vi "Handle Picture Key Down Event.vi"(7 "VKey":T1, 8 "error in (no error)":errorcluster, 11 "dialog info in":T2={"steering frame ref"=refnum, "active wheel indexes"=[], "FP Refs"={"VI Refnum"=refnum, "Menu Ref"=refnum, "Sub Panel"=refnum, "picture"=refnum, "Steering Type"=refnum, "zoom in"=refnum, "zoom out"=refnum, "zoom extents"=refnum, "Wheels"=refnum, "Add Wheel"=refnum, "Remove Wheel"=refnum, "Copy Wheel"=refnum, "Angle Units"=refnum}, "subpanel info"={"subpanel VI refs"=[], "subpanel types"=[], "main to subpanel command events"=[]}, "picture dragging state"={"dragging"=FALSE, "wheel index"=-1, "dragging mode"=enum."translate", "wheel start position"={"x"=0.0, "y"=0.0, "theta"=0.0}, "relative mouse position"={"x"=0.0, "y"=0.0}, "relative mouse init angle (rad)"=0.0}, "picture size (pixels)"={"Width"=500, "Height"=500}, "picture grid"=bytes[0], "click zones group"={"click zones array"=[], "num click zones"=0}, "draw options"={"draw wheel states?"=FALSE, "highlight wheel index"=-1, "pixels per unit"=10.0, "draw forward velocity?"=FALSE, "velocity scale"=1.0}}) -> (0 "error out":errorcluster, 1 "discard?":bool, 3 "dialog info out":T2={"steering frame ref"=refnum, "active wheel indexes"=[], "FP Refs"={"VI Refnum"=refnum, "Menu Ref"=refnum, "Sub Panel"=refnum, "picture"=refnum, "Steering Type"=refnum, "zoom in"=refnum, "zoom out"=refnum, "zoom extents"=refnum, "Wheels"=refnum, "Add Wheel"=refnum, "Remove Wheel"=refnum, "Copy Wheel"=refnum, "Angle Units"=refnum}, "subpanel info"={"subpanel VI refs"=[], "subpanel types"=[], "main to subpanel command events"=[]}, "picture dragging state"={"dragging"=FALSE, "wheel index"=-1, "dragging mode"=enum."translate", "wheel start position"={"x"=0.0, "y"=0.0, "theta"=0.0}, "relative mouse position"={"x"=0.0, "y"=0.0}, "relative mouse init angle (rad)"=0.0}, "picture size (pixels)"={"Width"=500, "Height"=500}, "picture grid"=bytes[0], "click zones group"={"click zones array"=[], "num click zones"=0}, "draw options"={"draw wheel states?"=FALSE, "highlight wheel index"=-1, "pixels per unit"=10.0, "draw forward velocity?"=FALSE, "velocity scale"=1.0}})   [LabVIEW 2017, in "NI_Robotics_Configure Steering Frame.lvlib"]
uses:
  <vilib>/robotics/Dialog/Configure Steering Frame/NI_Robotics_Configure Steering Frame.lvlib
  <vilib>/robotics/Dialog/Configure Steering Frame/Dialog Info.ctl
  <vilib>/robotics/Steering/Steering Frame/NI_Robotics_Steering Frame.lvclass
  <vilib>/robotics/Dialog/Configure Steering Frame/FP Refs.ctl
  <vilib>/robotics/Dialog/Configure Steering Frame/Subpanel Info.ctl
  <vilib>/robotics/Dialog/Configure Steering Frame/Main to Subpanel Command Event.ctl
  <vilib>/robotics/Dialog/Configure Steering Frame/Main to Subpanel Command.ctl
  <vilib>/robotics/Dialog/Configure Steering Frame/Dragging State.ctl
  <vilib>/robotics/Dialog/Configure Steering Frame/Dragging Mode.ctl
  <vilib>/Utility/miscctls.llb/LVBoundsTypeDef.ctl
  <vilib>/robotics/Dialog/Configure Steering Frame/Click Zone.ctl
  <vilib>/robotics/Utilities/Visualization/Steering Visualization/Steering Picture/Draw Steering Frame Options.ctl
  <vilib>/event_ctls.llb/eventvkey.ctl
  <vilib>/robotics/Utilities/Visualization/Steering Visualization/Steering Picture/NI_Robotics_Steering Picture.lvlib
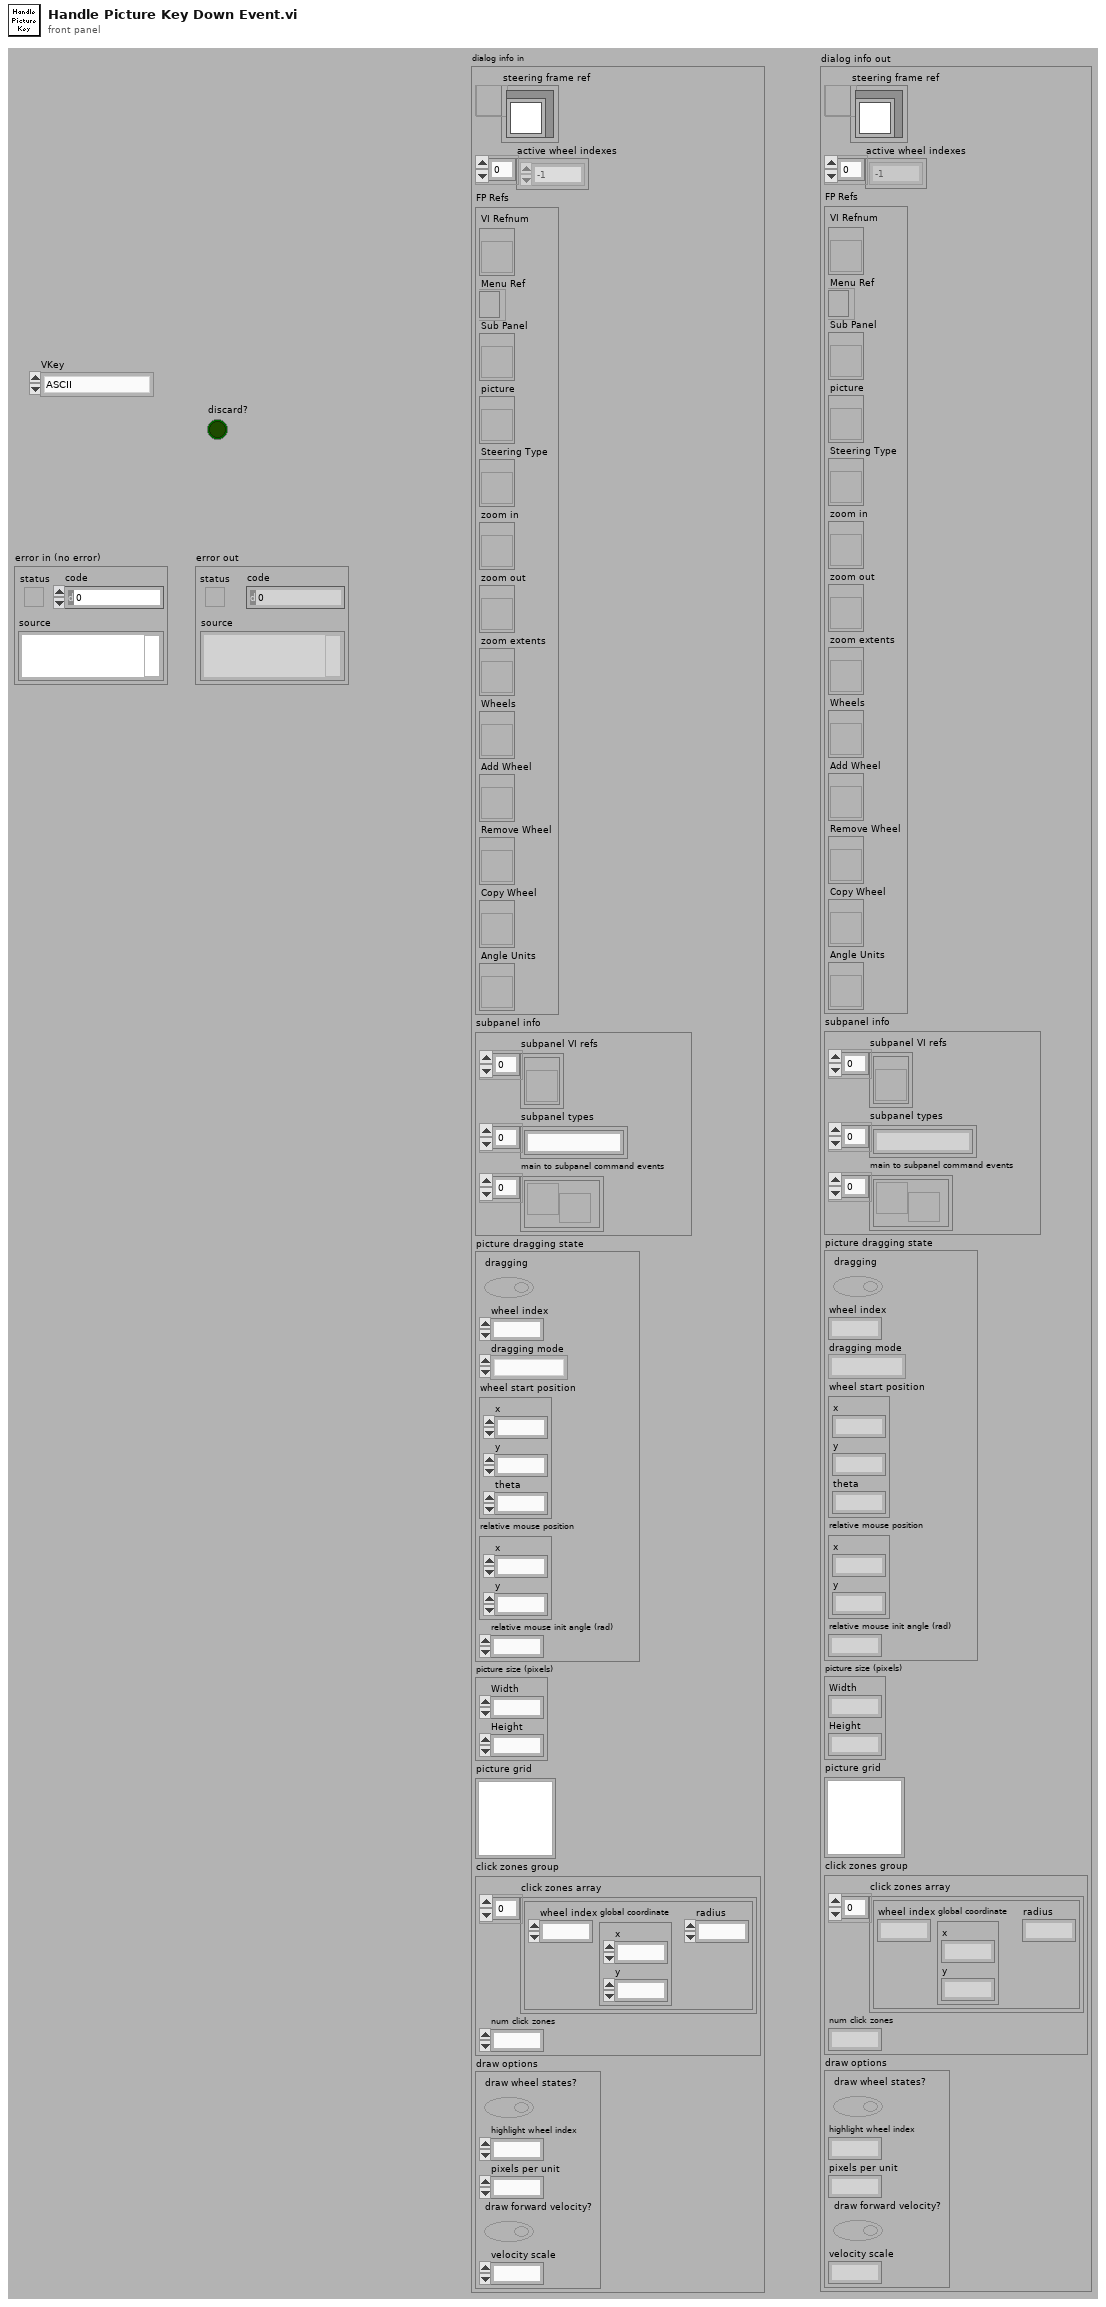
[diagram p1: front panel]
types:
  T1 = typedef "eventvkey.ctl" = enum16{"ASCII", "Enter", "Return", "Shift", "Ctrl", "Alt", "Cmd", "Opt", "Caps", "NumLock", "Clear", "Break", "Up", "Down", "Left", "Right", "Insert", "Delete", "Home", "End", "PageUp", "PageDown", "Escape", "Help", "Pause", "ScrollLock", "F1", "F2", "F3", "F4", "F5", "F6", "F7", "F8", "F9", "F10", "F11", "F12", "F13", "F14", "F15", "F16", "F17", "F18", "F19", "F20", "F21", "F22", "F23", "F24", "Play", "VolumeUp", "VolumeDown", "Mute", "Two Byte Char"}
  T2 = typedef "NI_Robotics_Configure Steering Frame.lvlib/Dialog Info.ctl" = cluster{"steering frame ref":refnum<data-value>, "active wheel indexes":i32[], "FP Refs":T3, "subpanel info":T4, "picture dragging state":T6, "picture size (pixels)":T8, "picture grid":picture, "click zones group":cluster{"click zones array":T9[], "num click zones":i32}, "draw options":T10}
  T3 = typedef "NI_Robotics_Configure Steering Frame.lvlib/FP Refs.ctl" = cluster{"VI Refnum":refnum<vi>, "Menu Ref":refnum<k9>, "Sub Panel":refnum<vi>, "picture":refnum<vi>, "Steering Type":refnum<vi>, "zoom in":refnum<vi>, "zoom out":refnum<vi>, "zoom extents":refnum<vi>, "Wheels":refnum<vi>, "Add Wheel":refnum<vi>, "Remove Wheel":refnum<vi>, "Copy Wheel":refnum<vi>, "Angle Units":refnum<vi>}
  T4 = typedef "NI_Robotics_Configure Steering Frame.lvlib/Subpanel Info.ctl" = cluster{"subpanel VI refs":refnum<vi>[], "subpanel types":string[], "main to subpanel command events":T5[]}
  T5 = typedef "NI_Robotics_Configure Steering Frame.lvlib/Main to Subpanel Command Event.ctl" = refnum<user-event>
  T6 = typedef "NI_Robotics_Configure Steering Frame.lvlib/Dragging State.ctl" = cluster{"dragging":bool, "wheel index":i32, "dragging mode":T7, "wheel start position":cluster{"x":dbl, "y":dbl, "theta":dbl}, "relative mouse position":cluster{"x":dbl, "y":dbl}, "relative mouse init angle (rad)":dbl}
  T7 = typedef "NI_Robotics_Configure Steering Frame.lvlib/Dragging Mode.ctl" = enum16{"translate", "rotate"}
  T8 = typedef "LVBoundsTypeDef.ctl" = cluster{"Width":u32, "Height":u32}
  T9 = typedef "NI_Robotics_Configure Steering Frame.lvlib/Click Zone.ctl" = cluster{"wheel index":i32, "global coordinate":cluster{"x":dbl, "y":dbl}, "radius":dbl}
  T10 = typedef "NI_Robotics_Steering Picture.lvlib/Draw Steering Frame Options.ctl" = cluster{"draw wheel states?":bool, "highlight wheel index":i32, "pixels per unit":dbl, "draw forward velocity?":bool, "velocity scale":dbl}
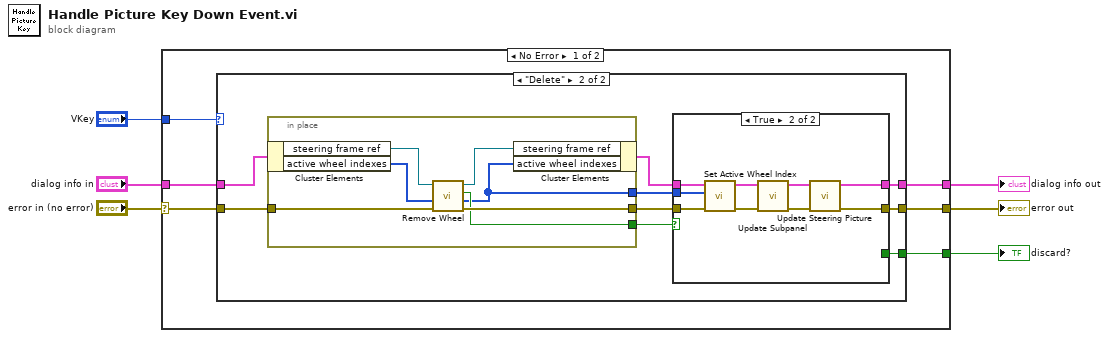
[diagram p0: block diagram]
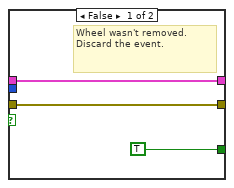
[diagram p3: hidden frame]
diagram:
  n1 = case shown="No Error" "error in (no error)" {
    selector: "error in (no error)" -> [w11 w44]
    tunnel: [w10 w44] -> w5
    tunnel: "dialog info in" -> [w9 w43]
    tunnel: [w8 w43] -> w3
    tunnel: "VKey" -> [w12 _]
    tunnel: [w7 _] -> w1
    frame No Error {
      n2 = case shown="\"Delete\"" w12 {
        tunnel: w11 -> [w14 w22]
        tunnel: [w14 w18] -> w10
        tunnel: w9 -> [w13 w23]
        tunnel: [w13 w19] -> w8
        tunnel: [_ w16] -> w7
        frame Default {
        }
        frame "Delete" {
          n3 = in-place {
            in-place-border: w22 -> [w39]
            in-place-border: [w38] -> w20
            in-place-border: [w37] -> w17
            in-place-border: [w36] -> w15
            n4 = in-place-cluster #1(w23) -> ("steering frame ref"=w42:refnum<data-value>, "active wheel indexes"=w41:i32[])
            n5 = call <vilib>:"Remove Wheel.vi"("error in (no error)"=w39, "active wheel indexes in"=w41, "steering frame ref in"=w42) -> ("error out"=w38:errorcluster, "active wheel indexes out"=w36:i32[], "removed?"=w37:bool, "steering frame ref out"=w40:refnum<data-value>)  [unwired: 5 in]
            n6 = in-place-cluster #1("steering frame ref"=w40, "active wheel indexes"=w36) -> (w21:T2)
          }
          n7 = case shown="True" w17 {
            tunnel: w21 -> [w26 w31]
            tunnel: w20 -> [w25 w29]
            tunnel: [w26 w34] -> w19
            tunnel: [w25 w32] -> w18
            tunnel: [TRUE _] -> w16
            tunnel: w15 -> [_ w27]
            frame False {
              # "Wheel wasn't removed.  Discard the event."
            }
            frame True {
              n8 = call <vilib>:"Set Active Wheel Index.vi"("error in (no error)"=w29, "active wheel indexes"=w27, "dialog info in"=w31) -> ("error out"=w28:errorcluster, "dialog info out"=w30:T2)  [unwired: 7 in]
              n9 = call <vilib>:"Update Subpanel.vi"("error in (no error)"=w28, "dialog info in"=w30) -> ("error out"=w33:errorcluster, "dialog info out"=w35:T2)  [unwired: 8 in]
              n10 = call <vilib>:"Update Steering Picture.vi"("error in (no error)"=w33, "dialog info in"=w35) -> ("error out"=w32:errorcluster, "dialog info out"=w34:T2)  [unwired: 8 in]
            }
          }
        }
      }
    }
    frame Error {
    }
  }
  "dialog info out" <- w3
  "error out" <- w5
  "discard?" <- w1
